vi "WPI_CameraPrint Error To Image.vi"(8 "error in (no error)":errorcluster, 9 "String":string, 11 "Image":T1) -> (2 "flattened error string":string, 3 "Image out":T1(plugin-control))   [LabVIEW 2017]
doc: "If there is an error, annotate the image to display the error code in the image display. Then check for the string. Otherwise pass the image through."
uses:
  <vilib>/vision/Image Controls.llb/IMAQ Image.ctl
  <vilib>/vision/NI_Vision_Development_Module.lvlib
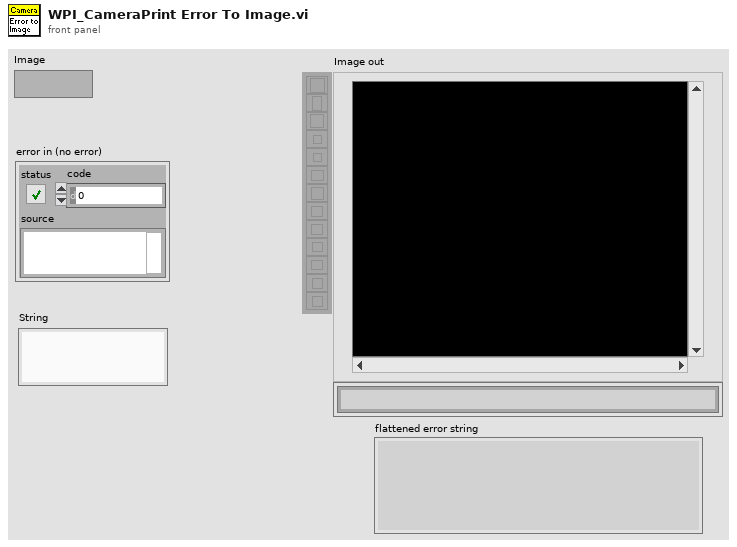
[diagram p1: front panel]
types:
  T1 = typedef "IMAQ Image.ctl" = refnum<image>
  T2 = cluster{"Desired Font (Application)":enum16{"User-specified Font", "Application Font", "System Font", "Dialog Font"}, "[User-specified Font]":cluster{"Font Name":string, "Size":i16, "Strikeout?":bool, "Italic?":bool, "Underline?":bool, "Outline?":bool, "Shadow?":bool, "Bold?":bool, "Rotation Angle":dbl}, "Horizontal Alignment":i16, "Vertical Alignment":i16}
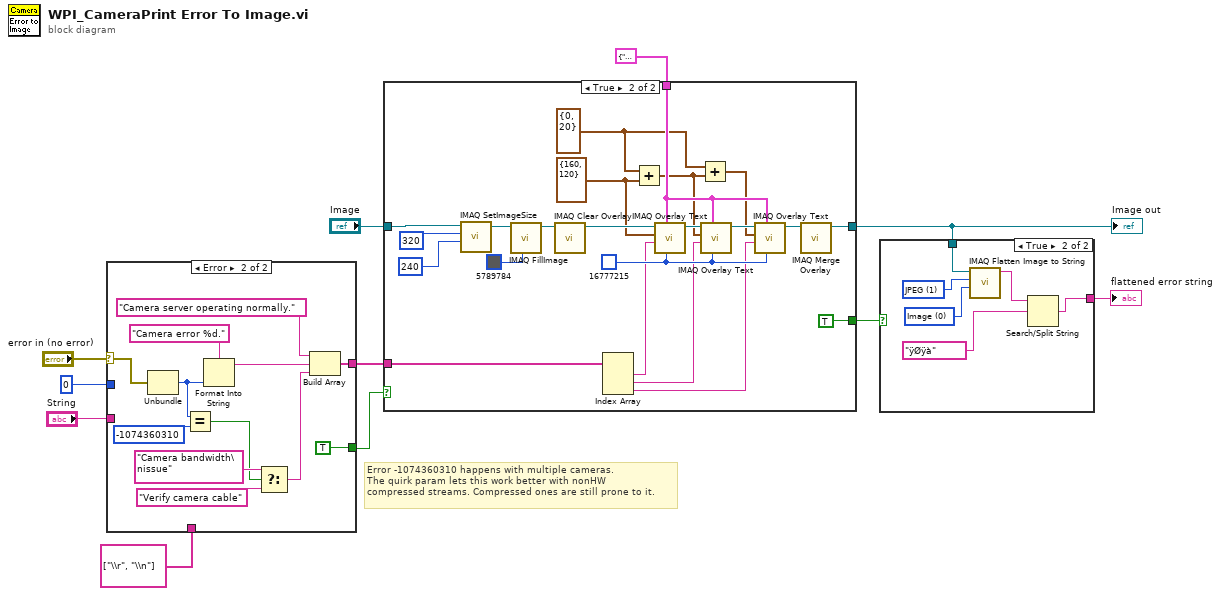
[diagram p0: block diagram]
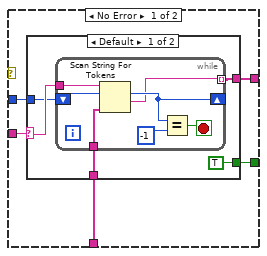
[diagram p2: hidden frame]
diagram:
  # "Error -1074360310 happens with multiple cameras.\nThe quirk param lets this work better with nonHW\ncompressed streams. Compressed ones are still prone to it."
  n1 = case shown="Error" "error in (no error)" {
    selector: "error in (no error)" -> [_ w40]
    tunnel: [w16 TRUE] -> w3
    tunnel: "String" -> [w15 _]
    tunnel: string[] ["\\r", "\\n"] ("delimiters (\\s,\\t,\\r,\\n)") -> [w14 _]
    tunnel: 0 -> [w13 _]
    tunnel: [w12 w36] -> w4
    frame No Error {
      n2 = case shown="Default" w15 {
        selector: w15 -> [w20 _]
        tunnel: [TRUE _] -> w16
        tunnel: w14 -> [w19 _]
        tunnel: w13 -> [w18 _]
        tunnel: [w17 _] -> w12
        frame Default {
          n3 = while {
            shift-right: [w25] -> _
            shift-left: w18 -> [w27]
            tunnel: w20 -> [w28]
            tunnel: w19 -> [w26]
            tunnel: [w22] -> w17 mode=indexing
            stop <- w23 stop-if-true
            n4 = Scan String For Tokens(6:w26, 8:w27, 9:w28) -> (1:w22:string, 2:w25:i32)  [unwired: 3 in, 2 out]
            n5 = Equal?(x=w25, y=-1) -> (x = y?=w23:bool)
          }
        }
        frame "" {
        }
      }
    }
    frame Error {
      n6 = Unbundle(w40) -> ("code"=w34:i32)  [unwired: 2 out]
      n7 = Equal?(x=w34, y=-1074360310) -> (x = y?=w29:bool)
      n8 = Format Into String(format string="Camera error %d.", w34) -> (resulting string=w38:string)  [unwired: 2 in, 1 out]
      n9 = Select(t="Camera bandwidth\nissue", s=w29, f="Verify camera cable") -> (s? t:f=w30:string)
      n10 = Build Array("Camera server operating normally.", w38, w30) -> (w36:string[])
    }
  }
  n11 = case shown="True" w3 {
    tunnel: "Image" -> [w41 w60]
    tunnel: [w41 w47] -> w7
    tunnel: T2 {"Desired Font (Application)"=enum."Application Font", "[User-specified Font]"={"Font Name"="", "Size"=12, "Strikeout?"=FALSE, "Italic?"=FALSE, "Underline?"=FALSE, "Outline?"=FALSE, "Shadow?"=FALSE, "Bold?"=FALSE, "Rotation Angle"=0.0}, "Horizontal Alignment"=1, "Vertical Alignment"=2} ("Font, Size & Style") -> [_ w53]
    tunnel: [_ TRUE] -> w2
    tunnel: w4 -> [_ w45]
    frame False {
    }
    frame True {
      w50 = cluster{"X":i32, "Y":i32} {"X"=0, "Y"=20} ("Origin")
      w52 = u32 16777215 ("Text Color (black)")
      w51 = cluster{"X":i32, "Y":i32} {"X"=160, "Y"=120} ("Origin")
      n12 = call "IMAQ SetImageSize"("Y Resolution"=240, "X Resolution"=320, "Image"=w60) -> ("Image Out"=w57:T1)  [unwired: 2 in, 1 out]
      n13 = call "IMAQ FillImage"("Color Pixel Value"=u32 5789784, "Image"=w57) -> ("Image Out"=w63:T1)  [unwired: 8 in, 1 out]
      n14 = call "IMAQ Clear Overlay"("Image"=w63) -> ("Image Out"=w62:T1)  [unwired: 9 in, 1 out]
      n15 = Index Array(array=w45) -> (element #1=w44:string, element #2=w43:string, element #3=w42:string)  [unwired: 3 in]
      n16 = Add(x=w50, y=w51) -> (x+y=w48:cluster{"X":i32, "Y":i32})
      n17 = call "IMAQ Overlay Text"("Text Color (black)"=w52, "Font, Size & Style"=w53, "String"=w44, "Origin"=w51, "Image"=w62) -> ("Image Out"=w56:T1)  [unwired: 5 in, 1 out]
      n18 = Add(x=w50, y=w48) -> (x+y=w49:cluster{"X":i32, "Y":i32})
      n19 = call "IMAQ Overlay Text"("Text Color (black)"=w52, "Font, Size & Style"=w53, "String"=w43, "Origin"=w48, "Image"=w56) -> ("Image Out"=w55:T1)  [unwired: 5 in, 1 out]
      n20 = call "IMAQ Overlay Text"("Text Color (black)"=w52, "Font, Size & Style"=w53, "String"=w42, "Origin"=w49, "Image"=w55) -> ("Image Out"=w54:T1)  [unwired: 5 in, 1 out]
      n21 = call "IMAQ Merge Overlay"("Image Src"=w54) -> ("Image Dst Out"=w47:T1)  [unwired: 9 in, 1 out]
    }
  }
  "Image out" <- w7
  n22 = case shown="True" w2 {
    tunnel: w7 -> [_ w65]
    tunnel: [_ w64] -> w10
    frame False {
    }
    frame True {
      w67 = 0 items=["Image", "Image and Vision Info", "Reference to Image"] ("Type of Flatten (Image and Vision Info)")
      w66 = 1 items=["None", "JPEG", "PACKED BINARY"] ("Compression (None)")
      n23 = call "IMAQ Flatten Image to String"("Type of Flatten (Image and Vision Info)"=w67, "Compression (None)"=w66, "Image"=w65) -> ("Data String"=w69:string)  [unwired: 7 in, 1 out]
      n24 = Search/Split String(string=w69, search string/char (-)="ÿØÿà" ("format string")) -> (match + rest of string=w64:string)  [unwired: 1 in, 2 out]
    }
  }
  "flattened error string" <- w10
